vi "Instrument Name and Icon UI.vi"() -> ()   [LabVIEW 2019]
uses:
  <vilib>/LabVIEW Icon API/lv_icon/Classes/Icon/Icon.lvclass
  <vilib>/LabVIEW Icon API/LabVIEW Icon API.lvlib
panel:
  in  "Launch Icon Editor":bool
  in  "Cancel":bool
  out "Instrument UI Library Icon":picture
  out "Instrument Library Icon":picture
  in  "OK":bool
  in  "Replace Template":string="[Rename]"
  in  "Icon Text":string="CYPHR"
  in  "Name":string="NewInstrument"
  in  "Instrument UI Color":u32(colorbox)=12123647
  in  "Instrument UI Text Color":u32(colorbox)
  in  "Instrument Color":u32(colorbox)=6618880
  in  "Instrument Text Color":u32(colorbox)
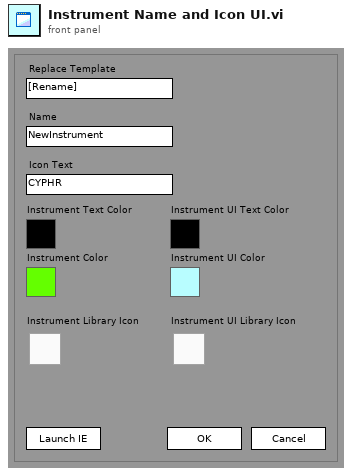
[diagram p1: front panel]
types:
  T1 = enum32{"Invalid", "Standard", "Closed", "Hidden", "Minimized", "Maximized"}
  T2 = enum32{"invalid app kind", "Development System", "Run Time System", "Student Edition", "Embedded LabVIEW", "Evaluation", "Custom"}
  T3 = cluster{"Core":cluster{"Current VI Reference":refnum<vi>, "Close Panel on Exit?":bool}, "Icon Text":string, "Instrument Text Color":u32, "Instrument  Color":u32, "Instrument UI Text Color":u32, "Instrument UI Color":u32, "Icon":refnum<class "Icon.lvclass">}
  T4 = cluster{"Current VI Reference":refnum<vi>, "Close Panel on Exit?":bool}
  T5 = typedef "imagedata.ctl" = cluster{"image type":i32, "image depth":i32, "image":u8[], "mask":u8[], "colors":u32[], "Rectangle":cluster{"left":i16, "top":i16, "right":i16, "bottom":i16}}
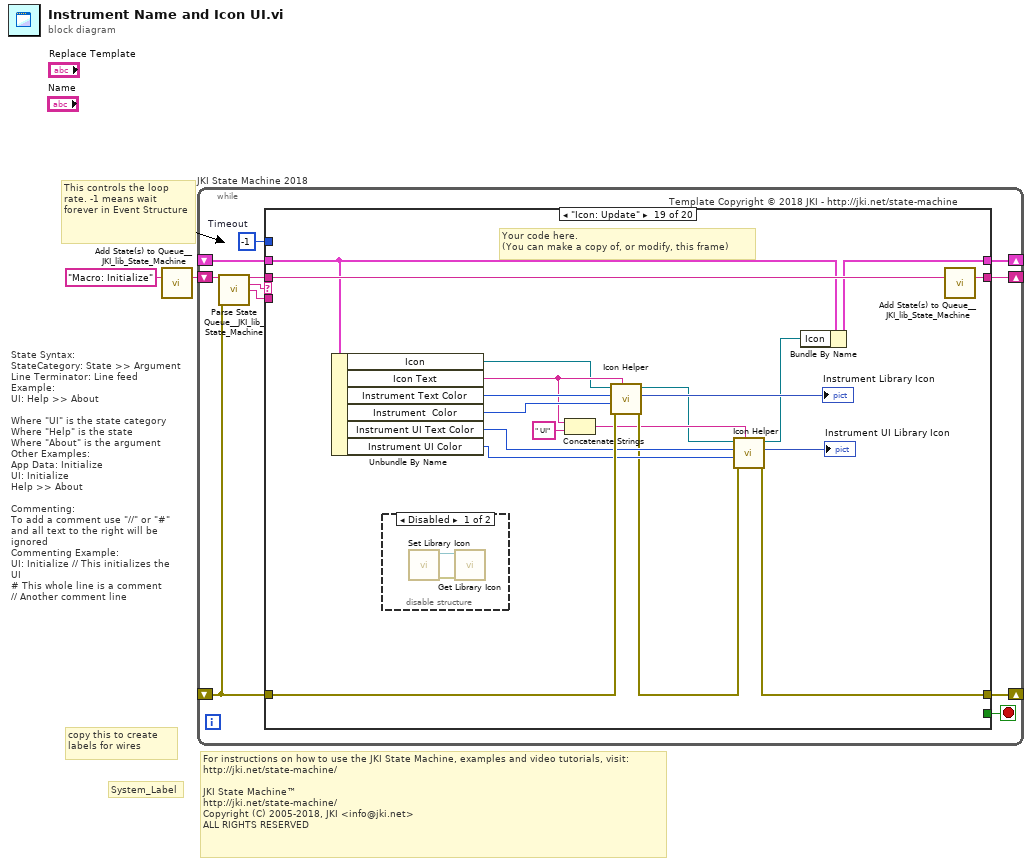
[diagram p0: block diagram]
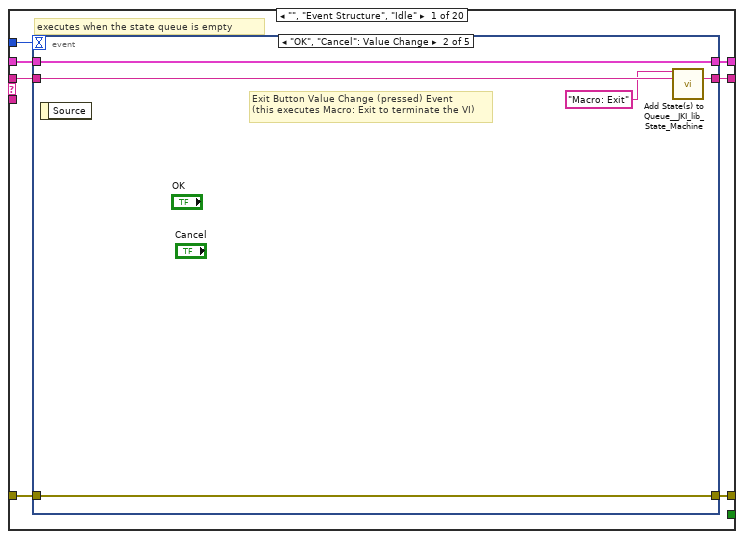
[diagram p2: hidden frame]
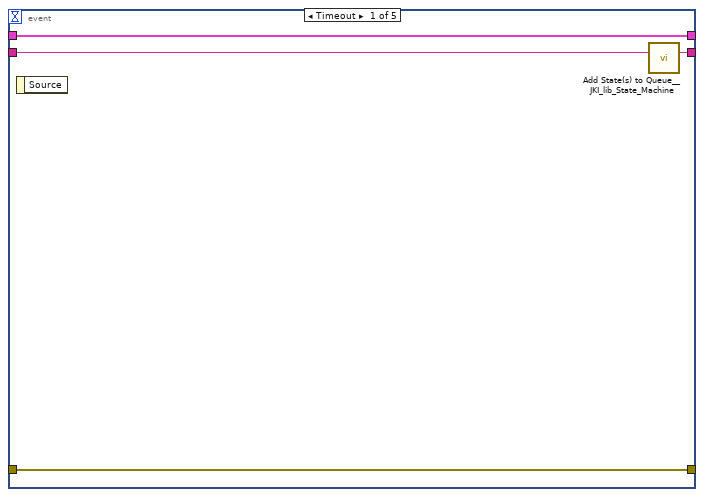
[diagram p3: hidden frame]
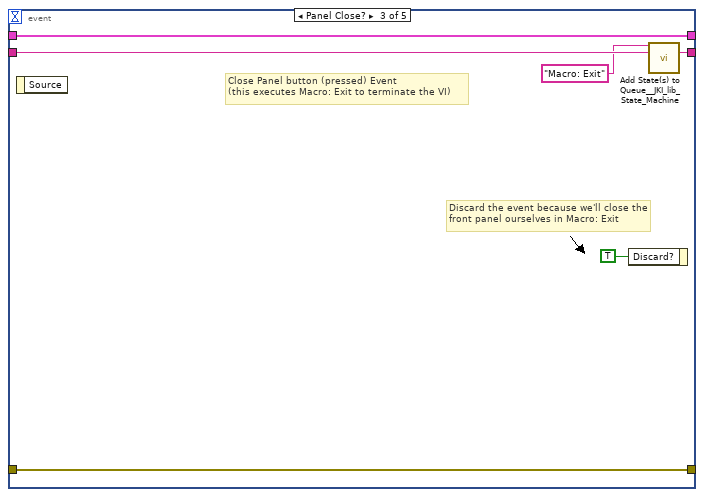
[diagram p4: hidden frame]
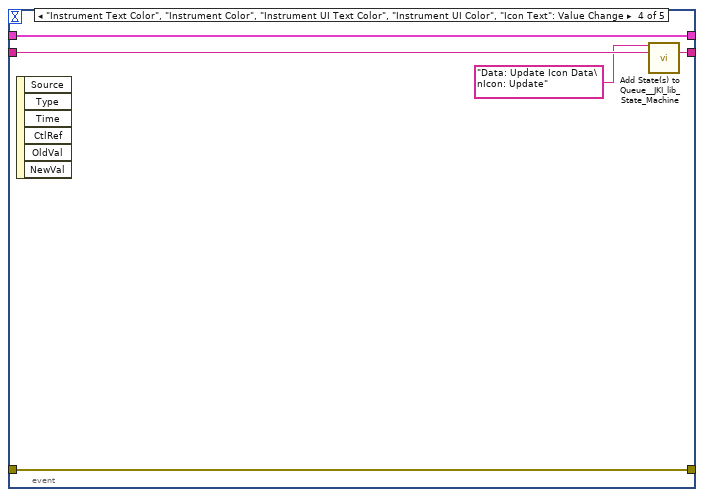
[diagram p5: hidden frame]
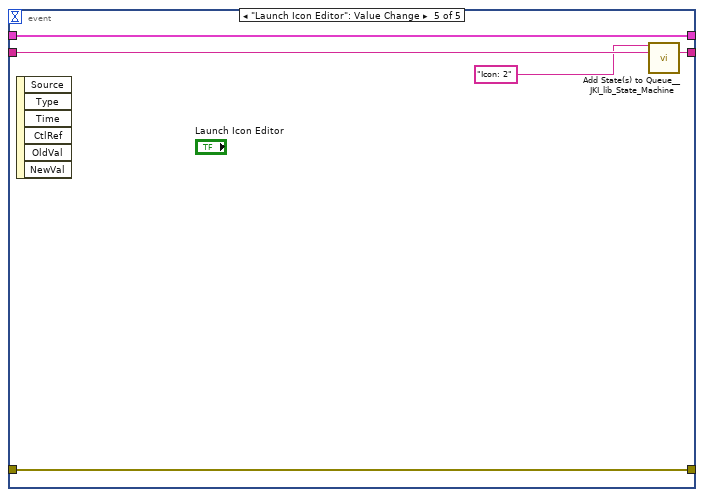
[diagram p6: hidden frame]
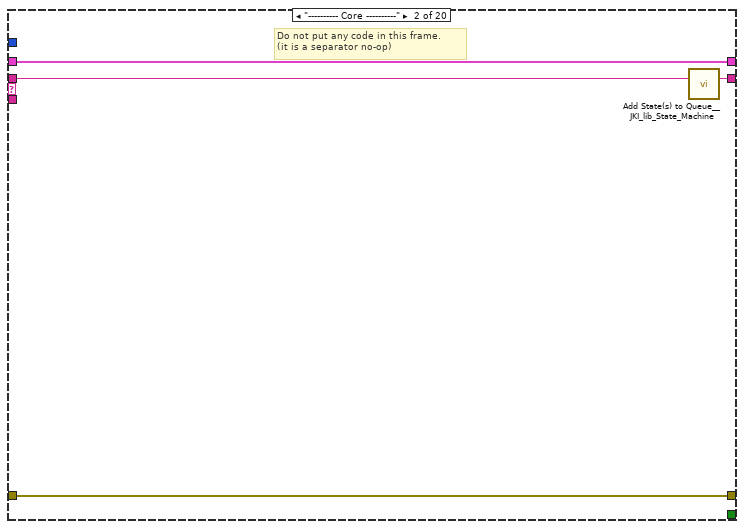
[diagram p7: hidden frame]
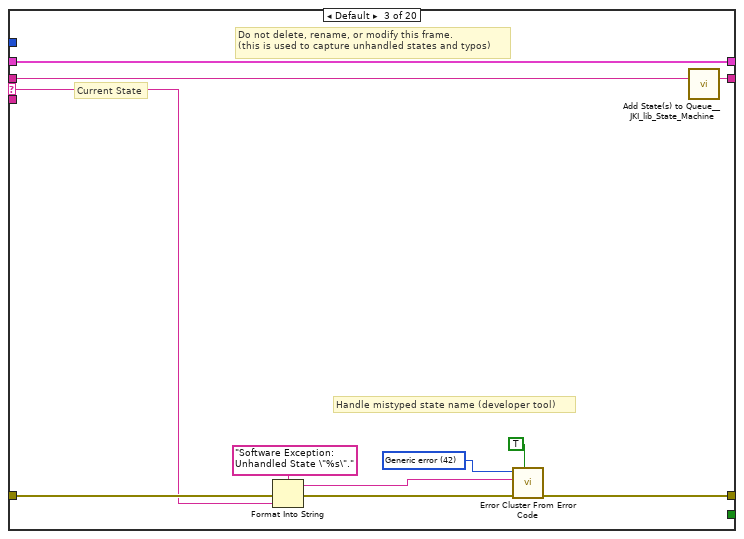
[diagram p8: hidden frame]
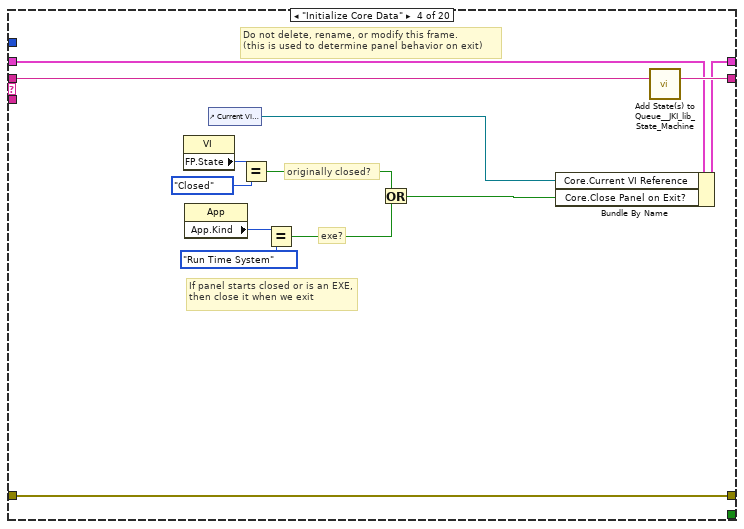
[diagram p9: hidden frame]
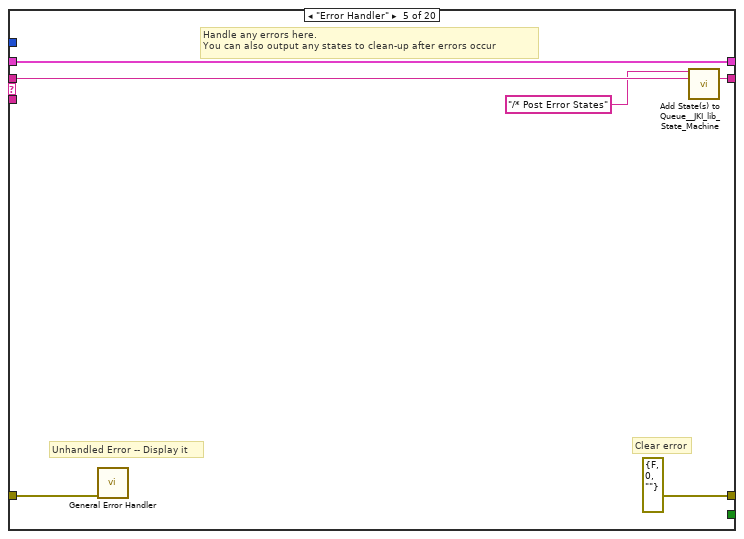
[diagram p10: hidden frame]
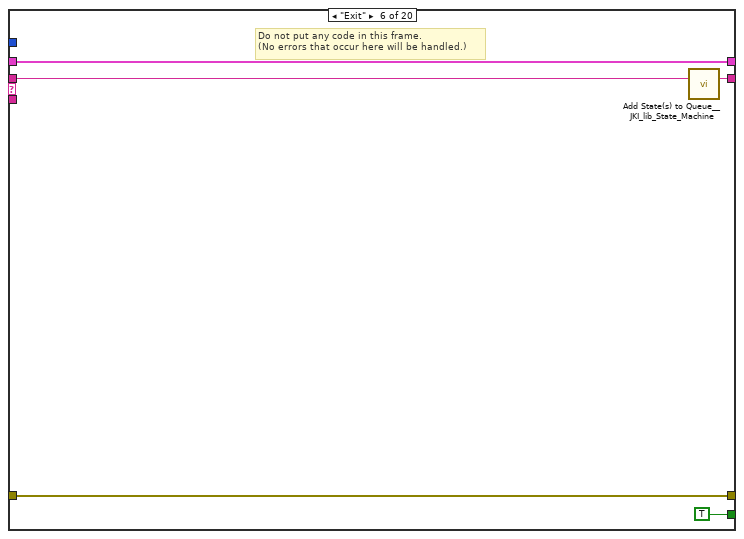
[diagram p11: hidden frame]
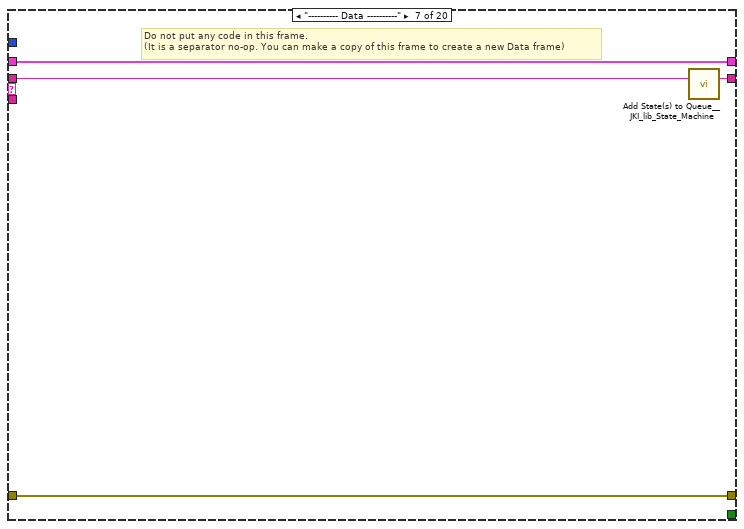
[diagram p12: hidden frame]
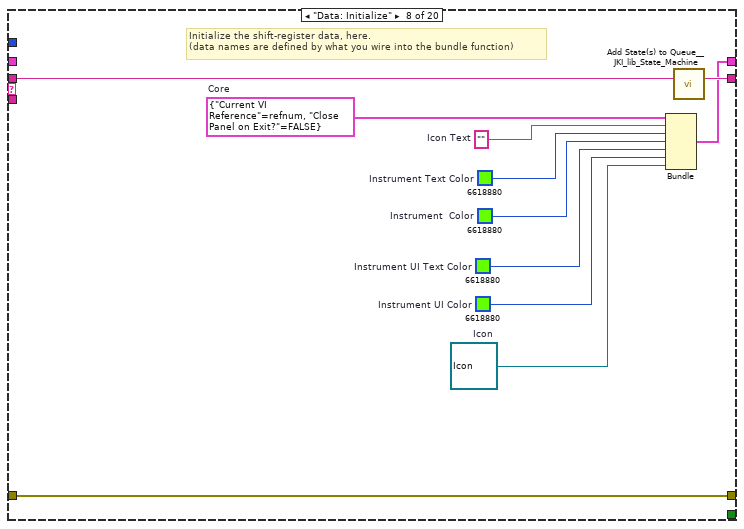
[diagram p13: hidden frame]
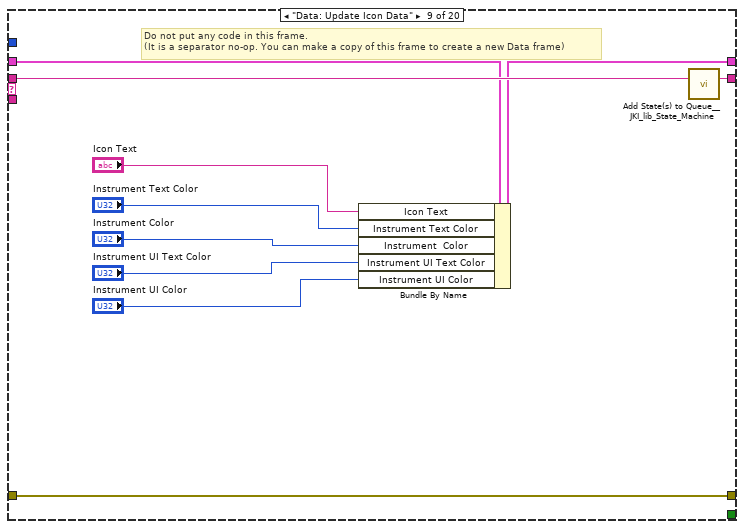
[diagram p14: hidden frame]
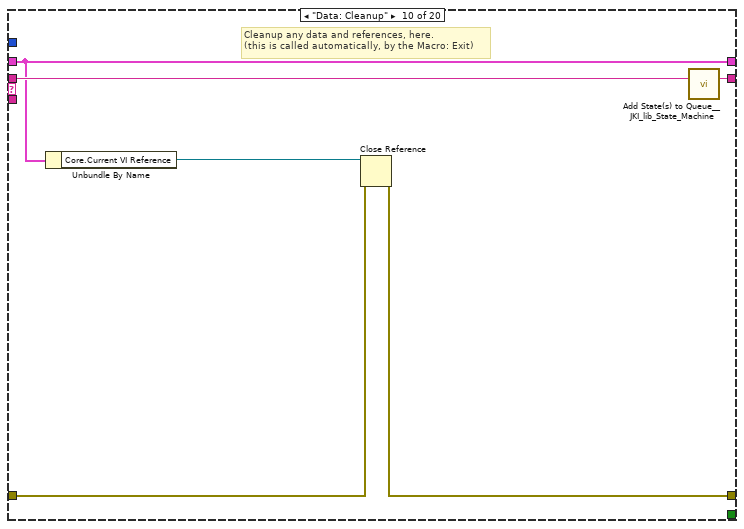
[diagram p15: hidden frame]
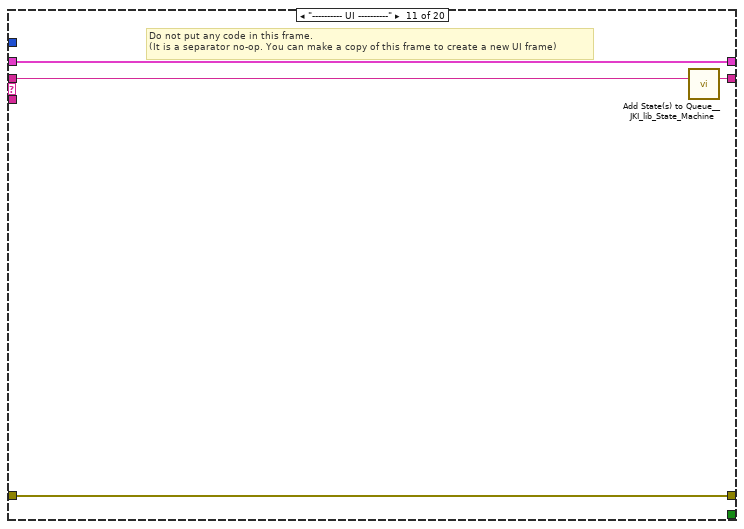
[diagram p16: hidden frame]
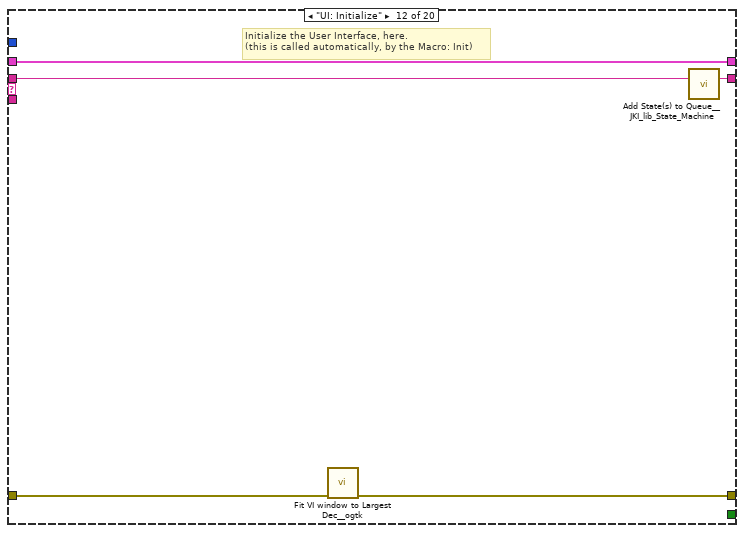
[diagram p17: hidden frame]
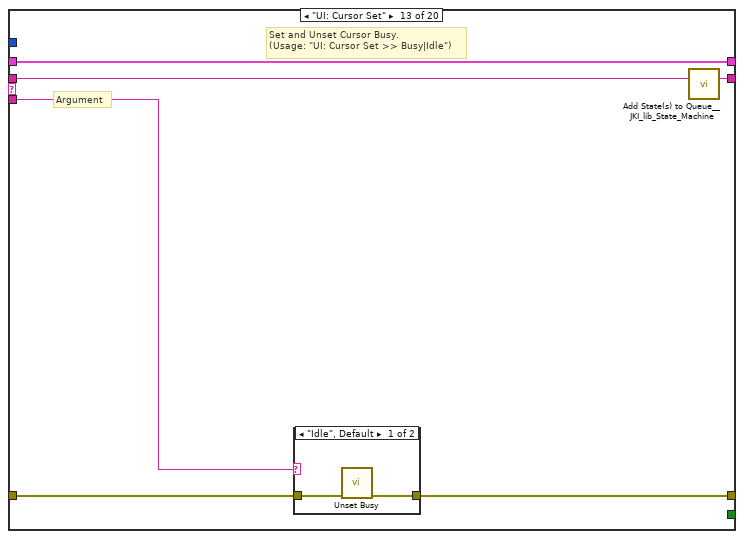
[diagram p18: hidden frame]
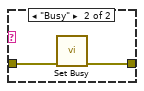
[diagram p19: hidden frame]
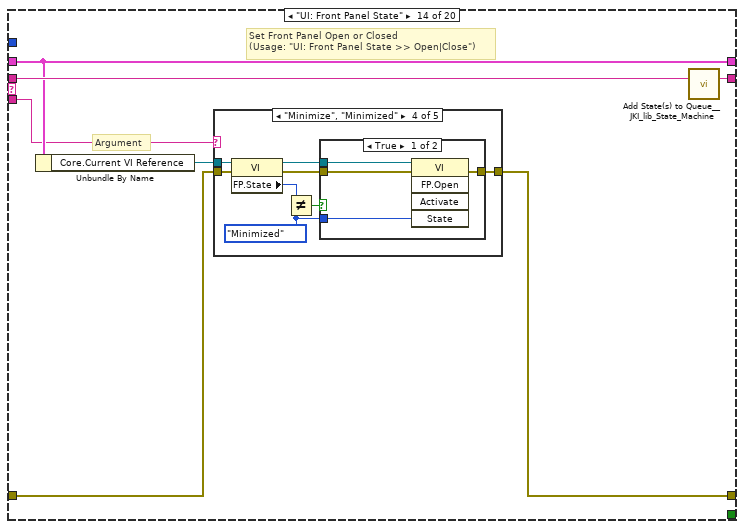
[diagram p20: hidden frame]
diagram:
  # "For instructions on how to use the JKI State Machine, examples and video tutorials, visit:\nhttp://jki.net/state-machine/\n\nJKI State Machine™\nhttp://jki.net/state-machine/\nCopyright (C) 2005-2018, JKI <info@jki.net>\nALL RIGHTS RESERVED"
  # "State Syntax:\nStateCategory: State >> Argument\nLine Terminator: Line feed\nExample:\nUI: Help >> About\n\nWhere \"UI\" is the state category\nWhere \"Help\" is the state\nWhere \"About\" is the argument\nOther Examples:\nApp Data: Initialize\nUI: Initialize\nHelp >> About\n\nCommenting:\nTo add a comment use \"//\" or \"#\" and all text to the right will be ignored\nCommenting Example:\nUI: Initialize // This initializes the UI\n# This whole line is a comment\n// Another comment line"
  # "copy this to create labels for wires"
  # "This controls the loop rate. -1 means wait forever in Event Structure"
  # "System_Label"
  n1 = call <vilib>:"Add State(s) to Queue__JKI_lib_State_Machine.vi"("State(s) in (\"\")"="Macro: Initialize") -> ("States Out"=w2:string)  [unwired: 14 in]
  n2 = while "JKI State Machine 2018" {
    shift-right: [w6] -> _
    shift-left: _ -> [w5]
    shift-right: [w9] -> _
    shift-left: _ -> [w3]
    shift-right: [w8] -> _
    shift-left: w2 -> [w10]
    stop <- w7 stop-if-true
    w4 = -1  # Timeout
    # "Template Copyright © 2018 JKI - http://jki.net/state-machine"
    n3 = call <vilib>:"Parse State Queue__JKI_lib_State_Machine.vi"("State Queue"=w10, "Error In (no error)"=w3) -> ("Remaining States"=w12:string, "Current State"=w13:string, "Arguments"=w11:string)  [unwired: 11 in]
    n4 = case shown="\"Icon: Update\"" w13 {
      selector: w13 -> [_ _ w50 _ _ _ _ _ _ _ _ _ _ _ _ _ _ _ _ _]
      tunnel: w12 -> [w20 w49 w54 w73 w79 w84 w88 w99 w109 w115 w119 w124 w130 w141 w210 w215 w225 w229 w248 w261]
      tunnel: w11 -> [_ _ _ _ _ _ _ _ _ _ _ _ w125 w135 _ _ _ _ _ _]
      tunnel: w5 -> [w18 w46 w52 w66 w76 w82 w85 _ w101 w110 w116 w122 w128 w137 w207 w212 w222 w226 w230 w256]
      tunnel: [w17 w47 w56 w70 errorcluster {"status"=FALSE, "code"=0, "source"=""} ("error out") w81 w86 w96 w107 w111 w117 w121 w126 w138 w208 w213 w223 w227 w239 w252] -> w9
      tunnel: w3 -> [w16 w47 w55 w70 w75 w81 w86 w96 w107 w112 w117 w120 w127 w139 w208 w213 w223 w227 w243 w258]
      tunnel: [w19 w48 w53 w72 w78 w83 w87 w98 w108 w114 w118 w123 w129 w140 w209 w214 w224 w228 w247 w260] -> w8
      tunnel: [_ _ _ _ _ TRUE _ _ _ _ _ _ _ _ _ _ _ _ _ _] -> w7
      tunnel: [w15 w46 w52 w71 w76 w82 w85 w97 w100 w110 w116 w122 w128 w137 w207 w212 w222 w226 w231 w257] -> w6
      tunnel: w4 -> [w14 _ _ _ _ _ _ _ _ _ _ _ _ _ _ _ _ _ _ _]
      frame "", "Event Structure", "Idle" {
        # "executes when the state queue is empty"
        n5 = event shown="[1] \"OK\", \"Cancel\": Value Change" {
          selector: _ -> [_ _ _ _ _]
          dyn-events: _ -> [_ _ _ _ _]
          timeout: w14 -> [_ _ _ _ _]
          tunnel: w20 -> [w24 w29 w35 w40 w45]
          tunnel: [w23 w28 w34 w39 w44] -> w19
          tunnel: w18 -> [w21 w26 w32 w36 w41]
          tunnel: [w22 w27 w33 w38 w43] -> w17
          tunnel: w16 -> [w22 w27 w33 w38 w43]
          tunnel: [w21 w26 w32 w36 w41] -> w15
          event Timeout {
            n6 = event-data() -> ()  [unwired: 1 in, 1 out]
            n7 = call <vilib>:"Add State(s) to Queue__JKI_lib_State_Machine.vi"("State(s) in (\"\")"=w24) -> ("States Out"=w23:string)  [unwired: 14 in]
          }
          event "OK", "Cancel": Value Change {
            # "Exit Button Value Change (pressed) Event\n(this executes Macro: Exit to terminate the VI)"
            n8 = event-data() -> ()  [unwired: 1 in, 1 out]
            n9 = call <vilib>:"Add State(s) to Queue__JKI_lib_State_Machine.vi"("State(s) in Front (\"\")"="Macro: Exit", "State(s) in (\"\")"=w29) -> ("States Out"=w28:string)  [unwired: 13 in]
          }
          event Panel Close? {
            # "Discard the event because we'll close the front panel ourselves in Macro: Exit"
            # "Close Panel button (pressed) Event\n(this executes Macro: Exit to terminate the VI)"
            n10 = event-data() -> ()  [unwired: 1 in, 1 out]
            n11 = event-data("Discard?"=TRUE) -> ()  [unwired: 1 in, 1 out]
            n12 = call <vilib>:"Add State(s) to Queue__JKI_lib_State_Machine.vi"("State(s) in Front (\"\")"="Macro: Exit", "State(s) in (\"\")"=w35) -> ("States Out"=w34:string)  [unwired: 13 in]
          }
          event "Instrument Text Color", "Instrument Color", "Instrument UI Text Color", "Instrument UI Color", "Icon Text": Value Change {
            n13 = event-data() -> ()  [unwired: 1 in, 6 out]
            n14 = call <vilib>:"Add State(s) to Queue__JKI_lib_State_Machine.vi"("State(s) in Front (\"\")"="Data: Update Icon Data\nIcon: Update", "State(s) in (\"\")"=w40) -> ("States Out"=w39:string)  [unwired: 13 in]
          }
          event "Launch Icon Editor": Value Change {
            n15 = event-data() -> ()  [unwired: 1 in, 6 out]
            n16 = call <vilib>:"Add State(s) to Queue__JKI_lib_State_Machine.vi"("State(s) in Front (\"\")"="Icon: 2", "State(s) in (\"\")"=w45) -> ("States Out"=w44:string)  [unwired: 13 in]
          }
        }
      }
      frame "---------- Core ----------" {
        # "Do not put any code in this frame.\n(it is a separator no-op)"
        n17 = call <vilib>:"Add State(s) to Queue__JKI_lib_State_Machine.vi"("State(s) in (\"\")"=w49) -> ("States Out"=w48:string)  [unwired: 14 in]
      }
      frame Default {
        w59 = 42 items=["No error", "Argument error", "Memory is full", "Out of zone", "End of file", "File already open", "Generic file I/O error", "File not found", "File permission error", "Disk is full", "Duplicate path", "Too many files open", "System feature not enabled", "Resource file not found", "Cannot add resource", "Resource not found", "Image not found", "Image memory error", "Pen does not exist", "Config type invalid", "Config token not found", "Config parse error", "Config memory error", "Bad external code format", "Bad external code offset", "External code not present", "Null window", "Destroy window error", "Null menu", "Print aborted", "Bad print record", "Print driver error", "Windows error during printing", "Memory error during printing", "Print dialog error", "Generic print error", "Invalid device refnum", "Device not found", "Device parameter error", "Device unit error", "Cannot open device", "Device call aborted", "Generic error", "Cancelled by user", "Object ID too low", "Object ID too high", "Object not in heap", "Unknown heap", "Unknown object (invalid DefProc)", "Unknown object (DefProc not in table)", "Message out of range", "Invalid (null) method", "Unknown message", "Manager call not supported", "Bad address", "Network operation in progress", "Network operation timed out", "Connection is busy", "Network attribute not supported", "Network error", "Address in use", "System out of memory", "Connection aborted", "Connection refused", "Not connected", "Already connected", "Connection closed", "Initialization error (interapplication manager)", "Bad occurrence", "Wait on unbound occurrence handler", "Occurrence queue overflow", "Datalog type conflict", "Unused", "Unrecognized type (interapplication manager)", "Memory corrupt", "Failed to make temporary DLL", "Old CIN version", "Drag socket not found", "Failed to load drop-object", "Failed to register OLE object", "Failed to release OLE object", "Format specifier type mismatch", "Unknown format specifier", "Too few format specifiers", "Too many format specifiers", "Scan failed", "Newer CIN version", "Error converting to variant", "Runtime menu error", "Password tampered", "Variant attribute not found", "Incompatible variant data type", "Event data is not available", "Event Store is not present", "Occurrence is not found", "Event Queue is not created", "Event info is not available", "Refnum passed is NULL", "Error retrieving Class GUID", "Error retrieving CoClass GUID", "Error retrieving TypeLib GUID.", "Bad built application magic bytes.", "Specific driver is different from the specific driver associated with the Logical Name.", "There is no session opened to the class driver.", "Max Error", "MAX - Error with config objects", "MAX - Error loading configuration", "MAX - Group not supported"]
        # "Current State"
        # "Do not delete, rename, or modify this frame.\n(this is used to capture unhandled states and typos)"
        # "Handle mistyped state name (developer tool)"
        n18 = Format Into String(format string="Software Exception: Unhandled State \"%s\"." ("message"), error in=w55, w50) -> (resulting string=w58:string, error out=w57:errorcluster)  [unwired: 1 in]
        n19 = call <vilib>:"Error Cluster From Error Code.vi"("show call chain? (False)"=TRUE, "error in (no error)"=w57, "error message (\"\")"=w58, "error code (0)"=w59) -> ("error out"=w56:errorcluster)  [unwired: 5 in]
        n20 = call <vilib>:"Add State(s) to Queue__JKI_lib_State_Machine.vi"("State(s) in (\"\")"=w54) -> ("States Out"=w53:string)  [unwired: 14 in]
      }
      frame "Initialize Core Data" {
        # "Do not delete, rename, or modify this frame.\n(this is used to determine panel behavior on exit)"
        # "originally closed?"
        # "exe?"
        # "If panel starts closed or is an EXE, then close it when we exit"
        n21 = property class="VI"() -> ("FP.State"=w63:T1)  [unwired: 2 in, 2 out]
        n22 = property class="App"() -> ("App.Kind"=w69:T2)  [unwired: 2 in, 2 out]
        n23 = control-ref of="Current VI Reference"() -> (w64:refnum<vi>)
        n24 = Equal?(x=w63, y=T1."Closed" ("Front Panel Window:State")) -> (x = y?=w61:bool)
        n25 = Equal?(x=w69, y=T2."Run Time System" ("Application:Kind")) -> (x = y?=w67:bool)
        n26 = Or(x=w61, y=w67) -> (x .or. y?=w65:bool)
        n27 = Bundle By Name(cluster=w66, "Core.Current VI Reference"=w64, "Core.Close Panel on Exit?"=w65) -> (w71:T3)
        n28 = call <vilib>:"Add State(s) to Queue__JKI_lib_State_Machine.vi"("State(s) in (\"\")"=w73) -> ("States Out"=w72:string)  [unwired: 14 in]
      }
      frame "Error Handler" {
        # "Unhandled Error -- Display it"
        # "Handle any errors here.\nYou can also output any states to clean-up after errors occur"
        # "Clear error"
        n29 = call <vilib>:"General Error Handler.vi"("error in (no error)"=w75) -> ()  [unwired: 10 in, 5 out]
        n30 = call <vilib>:"Add State(s) to Queue__JKI_lib_State_Machine.vi"("State(s) in Front (\"\")"="/* Post Error States", "State(s) in (\"\")"=w79) -> ("States Out"=w78:string)  [unwired: 13 in]
      }
      frame "Exit" {
        # "Do not put any code in this frame.\n(No errors that occur here will be handled.)"
        n31 = call <vilib>:"Add State(s) to Queue__JKI_lib_State_Machine.vi"("State(s) in (\"\")"=w84) -> ("States Out"=w83:string)  [unwired: 14 in]
      }
      frame "---------- Data ----------" {
        # "Do not put any code in this frame.\n(It is a separator no-op. You can make a copy of this frame to create a new Data frame)"
        n32 = call <vilib>:"Add State(s) to Queue__JKI_lib_State_Machine.vi"("State(s) in (\"\")"=w88) -> ("States Out"=w87:string)  [unwired: 14 in]
      }
      frame "Data: Initialize" {
        w89 = refnum<class "Icon.lvclass"> refnum  # Icon
        w90 = ""  # Icon Text
        w91 = u32 6618880  # Instrument UI Color
        w92 = u32 6618880  # Instrument UI Text Color
        w93 = u32 6618880  # Instrument  Color
        w94 = u32 6618880  # Instrument Text Color
        w95 = T4 {"Current VI Reference"=refnum, "Close Panel on Exit?"=FALSE}  # Core
        # "Initialize the shift-register data, here.\n(data names are defined by what you wire into the bundle function)"
        n33 = Bundle("Core"=w95, "Icon Text"=w90, "Instrument Text Color"=w94, "Instrument  Color"=w93, "Instrument UI Text Color"=w92, "Instrument UI Color"=w91, "Icon"=w89) -> (w97:T3)  [unwired: 1 in]
        n34 = call <vilib>:"Add State(s) to Queue__JKI_lib_State_Machine.vi"("State(s) in (\"\")"=w99) -> ("States Out"=w98:string)  [unwired: 14 in]
      }
      frame "Data: Update Icon Data" {
        # "Do not put any code in this frame.\n(It is a separator no-op. You can make a copy of this frame to create a new Data frame)"
        n35 = Bundle By Name(cluster=w101, "Icon Text"="Icon Text", "Instrument Text Color"="Instrument Text Color", "Instrument  Color"="Instrument Color", "Instrument UI Text Color"="Instrument UI Text Color", "Instrument UI Color"="Instrument UI Color") -> (w100:T3)
        n36 = call <vilib>:"Add State(s) to Queue__JKI_lib_State_Machine.vi"("State(s) in (\"\")"=w109) -> ("States Out"=w108:string)  [unwired: 14 in]
      }
      frame "Data: Cleanup" {
        # "Cleanup any data and references, here.\n(this is called automatically, by the Macro: Exit)"
        n37 = Unbundle By Name(w110) -> ("Core.Current VI Reference"=w113:refnum<vi>)
        n38 = Close Reference(reference=w113, error in (no error)=w112) -> (error out=w111:errorcluster)
        n39 = call <vilib>:"Add State(s) to Queue__JKI_lib_State_Machine.vi"("State(s) in (\"\")"=w115) -> ("States Out"=w114:string)  [unwired: 14 in]
      }
      frame "---------- UI ----------" {
        # "Do not put any code in this frame.\n(It is a separator no-op. You can make a copy of this frame to create a new UI frame)"
        n40 = call <vilib>:"Add State(s) to Queue__JKI_lib_State_Machine.vi"("State(s) in (\"\")"=w119) -> ("States Out"=w118:string)  [unwired: 14 in]
      }
      frame "UI: Initialize" {
        # "Initialize the User Interface, here.\n(this is called automatically, by the Macro: Init)"
        n41 = call <userlib>:"Fit VI window to Largest Dec__ogtk.vi"("error in (no error)"=w120) -> ("error out"=w121:errorcluster)  [unwired: 5 in, 1 out]
        n42 = call <vilib>:"Add State(s) to Queue__JKI_lib_State_Machine.vi"("State(s) in (\"\")"=w124) -> ("States Out"=w123:string)  [unwired: 14 in]
      }
      frame "UI: Cursor Set" {
        # "Argument"
        # "Set and Unset Cursor Busy.\n(Usage: \"UI: Cursor Set >> Busy|Idle\")"
        n43 = case shown="\"Idle\", Default" w125 {
          tunnel: w127 -> [w132 w134]
          tunnel: [w131 w133] -> w126
          frame "Idle", Default {
            n44 = call <vilib>:"Unset Busy.vi"("error in (no error)"=w132) -> ("error out"=w131:errorcluster)  [unwired: 10 in]
          }
          frame "Busy" {
            n45 = call <vilib>:"Set Busy.vi"("error in (no error)"=w134) -> ("error out"=w133:errorcluster)  [unwired: 9 in, 1 out]
          }
        }
        n46 = call <vilib>:"Add State(s) to Queue__JKI_lib_State_Machine.vi"("State(s) in (\"\")"=w130) -> ("States Out"=w129:string)  [unwired: 14 in]
      }
      frame "UI: Front Panel State" {
        # "Argument"
        # "Set Front Panel Open or Closed\n(Usage: \"UI: Front Panel State >> Open|Close\")"
        n47 = Unbundle By Name(w137) -> ("Core.Current VI Reference"=w136:refnum<vi>)
        n48 = case shown="\"Minimize\", \"Minimized\"" w135 {
          tunnel: w139 -> [w147 w162 w173 w186 w199]
          tunnel: [w149 w163 w175 w188 w201] -> w138
          tunnel: w136 -> [w148 w160 w174 w187 w200]
          frame "Open", "Standard", Default {
            w142 = T1."Standard" ("State")
            n49 = property class="VI"(reference=w148, error in=w147) -> (reference out=w145:refnum<vi>, error out=w146:errorcluster, "FP.State"=w144:T1)
            n50 = Not Equal?(x=w144, y=w142) -> (x != y?=w143:bool)
            n51 = case shown="True" w143 {
              tunnel: [w153 w155] -> w149
              tunnel: w146 -> [w152 w155]
              tunnel: w145 -> [w151 _]
              tunnel: w142 -> [w150 _]
              frame True {
                n52 = invoke class="VI" method="FP.Open"(reference=w151, error in=w152, "Activate"=TRUE, "State"=w150) -> (error out=w153:errorcluster)  [unwired: 1 in, 4 out]
              }
              frame False {
              }
            }
          }
          frame "Close", "Closed" {
            n53 = property class="VI"(reference=w160, error in=w162) -> (reference out=w159:refnum<vi>, error out=w161:errorcluster, "FP.State"=w157:T1)
            n54 = Not Equal?(x=w157, y=T1."Closed" ("Front Panel Window:State")) -> (x != y?=w156:bool)
            n55 = case shown="True" w156 {
              tunnel: [w164 w167] -> w163
              tunnel: w161 -> [w164 w166]
              tunnel: w159 -> [_ w165]
              frame False {
              }
              frame True {
                n56 = invoke class="VI" method="FP.Close"(reference=w165, error in=w166) -> (error out=w167:errorcluster)  [unwired: 1 in, 2 out]
              }
            }
          }
          frame "Hidden", "Hide" {
            w168 = T1."Hidden" ("State")
            n57 = property class="VI"(reference=w174, error in=w173) -> (reference out=w171:refnum<vi>, error out=w172:errorcluster, "FP.State"=w170:T1)
            n58 = Not Equal?(x=w170, y=w168) -> (x != y?=w169:bool)
            n59 = case shown="True" w169 {
              tunnel: [w179 w180] -> w175
              tunnel: w172 -> [w178 w180]
              tunnel: w171 -> [w177 _]
              tunnel: w168 -> [w176 _]
              frame True {
                n60 = invoke class="VI" method="FP.Open"(reference=w177, error in=w178, "State"=w176) -> (error out=w179:errorcluster)  [unwired: 2 in, 4 out]
              }
              frame False {
              }
            }
          }
          frame "Minimize", "Minimized" {
            w181 = T1."Minimized" ("State")
            n61 = property class="VI"(reference=w187, error in=w186) -> (reference out=w184:refnum<vi>, error out=w185:errorcluster, "FP.State"=w183:T1)
            n62 = Not Equal?(x=w183, y=w181) -> (x != y?=w182:bool)
            n63 = case shown="True" w182 {
              tunnel: [w192 w193] -> w188
              tunnel: w185 -> [w191 w193]
              tunnel: w184 -> [w190 _]
              tunnel: w181 -> [w189 _]
              frame True {
                n64 = invoke class="VI" method="FP.Open"(reference=w190, error in=w191, "State"=w189) -> (error out=w192:errorcluster)  [unwired: 2 in, 4 out]
              }
              frame False {
              }
            }
          }
          frame "Maximize", "Maximized" {
            w194 = T1."Maximized" ("State")
            n65 = property class="VI"(reference=w200, error in=w199) -> (reference out=w197:refnum<vi>, error out=w198:errorcluster, "FP.State"=w196:T1)
            n66 = Not Equal?(x=w196, y=w194) -> (x != y?=w195:bool)
            n67 = case shown="True" w195 {
              tunnel: [w205 w206] -> w201
              tunnel: w198 -> [w204 w206]
              tunnel: w197 -> [w203 _]
              tunnel: w194 -> [w202 _]
              frame True {
                n68 = invoke class="VI" method="FP.Open"(reference=w203, error in=w204, "State"=w202) -> (error out=w205:errorcluster)  [unwired: 2 in, 4 out]
              }
              frame False {
              }
            }
          }
        }
        n69 = call <vilib>:"Add State(s) to Queue__JKI_lib_State_Machine.vi"("State(s) in (\"\")"=w141) -> ("States Out"=w140:string)  [unwired: 14 in]
      }
      frame "---------- Macro ----------" {
        # "Do not put any code in this frame.\n(It is a separator no-op. You can make a copy of this frame to create a new Macro frame)"
        n70 = call <vilib>:"Add State(s) to Queue__JKI_lib_State_Machine.vi"("State(s) in (\"\")"=w210) -> ("States Out"=w209:string)  [unwired: 14 in]
      }
      frame "Macro: Initialize" {
        w211 = "Data: Initialize\nInitialize Core Data\nUI: Initialize\nUI: Front Panel State >> Open\nData: Update Icon Data\nIcon: Update"  # Data: Initialize Initialize Core Data UI: Initialize UI: Front Panel State >> Open Data: Update Icon Data Icon: Update
        # "Initialization Macro\n(This is called once, when the VI starts)"
        n71 = call <vilib>:"Add State(s) to Queue__JKI_lib_State_Machine.vi"("State(s) in Front (\"\")"=w211, "State(s) in (\"\")"=w215) -> ("States Out"=w214:string)  [unwired: 13 in]
      }
      frame "Macro: Exit" {
        # "Exit Macro\n(This is called once, when the VI exits)"
        n72 = Unbundle By Name(w222) -> ("Core.Close Panel on Exit?"=w221:bool)
        n73 = Select(t="UI: Front Panel State >> Close", s=w221, f="") -> (s? t:f=w218:string)
        n74 = call <vilib>:"Add State(s) to Queue__JKI_lib_State_Machine.vi"("State(s) in (\"\")"=w218, "State(s) at Back (\"\")"="Data: Cleanup\nExit") -> ("States Out"=w216:string)  [unwired: 13 in]
        n75 = call <vilib>:"Add State(s) to Queue__JKI_lib_State_Machine.vi"("State(s) in Front (\"\")"=w216, "State(s) in (\"\")"=w225) -> ("States Out"=w224:string)  [unwired: 13 in]
      }
      frame "---------- Icon ----------" {
        # "Template Separator\n(You can make a copy of, or modify, this frame)"
        n76 = call <vilib>:"Add State(s) to Queue__JKI_lib_State_Machine.vi"("State(s) in (\"\")"=w229) -> ("States Out"=w228:string)  [unwired: 14 in]
      }
      frame "Icon: Update" {
        # "Your code here.\n(You can make a copy of, or modify, this frame)"
        n77 = Unbundle By Name(w230) -> ("Icon"=w234:refnum<class "Icon.lvclass">, "Icon Text"=w238:string, "Instrument Text Color"=w246:u32, "Instrument  Color"=w245:u32, "Instrument UI Text Color"=w242:u32, "Instrument UI Color"=w241:u32)
        n78 = disable-structure shown="Disabled" {
          frame Disabled {
            n79 = call <vilib>:"Set Library Icon.vi"() -> ("error out"=w249:errorcluster, "Library Refnum out"=w250:refnum<vi>)  [unwired: 10 in]
            n80 = call <vilib>:"Get Library Icon.vi"("error in (no error)"=w249, "Library Refnum in"=w250) -> ()  [unwired: 7 in, 3 out]
          }
          frame Enabled {
          }
        }
        n81 = Concatenate Strings(w238, " UI" ("string")) -> (w237:string)
        n82 = call "Icon Helper.vi"("Icon Text"=w238, "error in (no error)"=w243, "Instrument  Color"=w245, "Instrument Text Color"=w246, "Icon.lvclass in"=w234) -> ("error out"=w240:errorcluster, "new picture"=→"Instrument Library Icon":picture, "lv_icon.lvlib:Icon.lvclass out"=w233:refnum<class "Icon.lvclass">)  [unwired: 4 in]
        n83 = call "Icon Helper.vi"("Icon Text"=w237, "error in (no error)"=w240, "Instrument  Color"=w241, "Instrument Text Color"=w242, "Icon.lvclass in"=w233) -> ("error out"=w239:errorcluster, "new picture"=→"Instrument UI Library Icon":picture, "lv_icon.lvlib:Icon.lvclass out"=w232:refnum<class "Icon.lvclass">)  [unwired: 4 in]
        n84 = Bundle By Name(cluster=w230, "Icon"=w232) -> (w231:T3)
        n85 = call <vilib>:"Add State(s) to Queue__JKI_lib_State_Machine.vi"("State(s) in (\"\")"=w248) -> ("States Out"=w247:string)  [unwired: 14 in]
      }
      frame "Icon: 2" {
        # "Your code here.\n(You can make a copy of, or modify, this frame)"
        n86 = Unbundle By Name(w256) -> ("Icon"=w259:refnum<class "Icon.lvclass">)
        n87 = call <vilib>:"Launch Icon Editor.vi"("error in (no error)"=w258, "Icon in"=w259) -> ("error out"=w253:errorcluster, "Icon out"=w254:refnum<class "Icon.lvclass">)  [unwired: 7 in, 1 out]
        n88 = call <vilib>:"Get Flattened Image.vi"("error in (no error)"=w253, "lv_icon.lvlib:Icon.lvclass in"=w254) -> ("error out"=w252:errorcluster, "Color Image"=w255:T5)  [unwired: 6 in, 2 out]
        n89 = Bundle By Name(cluster=w256, "Icon"=w254) -> (w257:T3)
        n90 = call <vilib>:"Draw Flattened Pixmap.vi"("image data"=w255) -> ("new picture"=w251:picture)  [unwired: 8 in]
        n91 = local write "Instrument Library Icon"(w251) -> ()
        n92 = call <vilib>:"Add State(s) to Queue__JKI_lib_State_Machine.vi"("State(s) in (\"\")"=w261) -> ("States Out"=w260:string)  [unwired: 14 in]
      }
    }
  }
